vi "CSP_updateCSP_Parameters.vi"(8 "error in (no error)":errorcluster, 10 "Indicators Ref":T1, 11 "CSP.lvclass":refnum<class "CSP.lvclass">) -> (0 "error out":errorcluster, 3 "output cluster":refnum<class "CSP.lvclass">)   [LabVIEW 2016, in "Spatial Pattern Filter.lvlib" / "CSP.lvclass"]
uses:
  CSP.lvclass
  CSP.lvclass/CSP.ctl
  Spatial Pattern Filter.lvlib
panel:
  # "This VI is a part of BCI Design library, http://www.ru-bci.org \nCopyright © 2020, Sotnikov Peter, All rights reserved. License: GNU GPLv3"
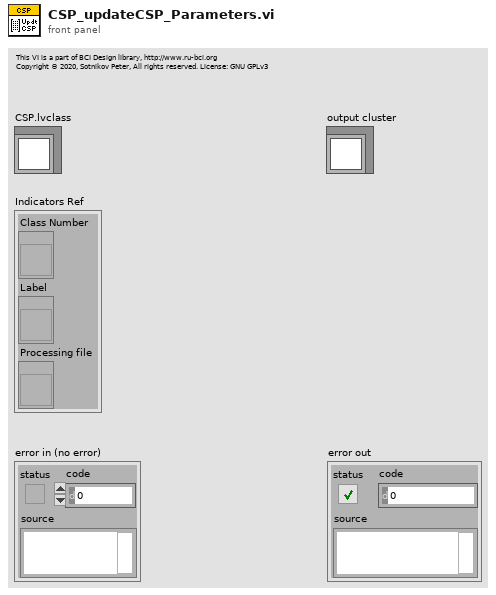
[diagram p1: front panel]
types:
  T1 = cluster{"Class Number":refnum<vi>, "Label":refnum<vi>, "Processing file":refnum<vi>}
  T2 = typedef "NI_Matrix.lvlib/RealMatrix.ctl" = dbl[][]
  T3 = cluster{"CSPMatrix":T2, "CovarianceMatrix1":T2, "CovarianceMatrix2":T2}[]
  T4 = cluster{"CSPMatrix":T2, "CovarianceMatrix1":T2, "CovarianceMatrix2":T2}
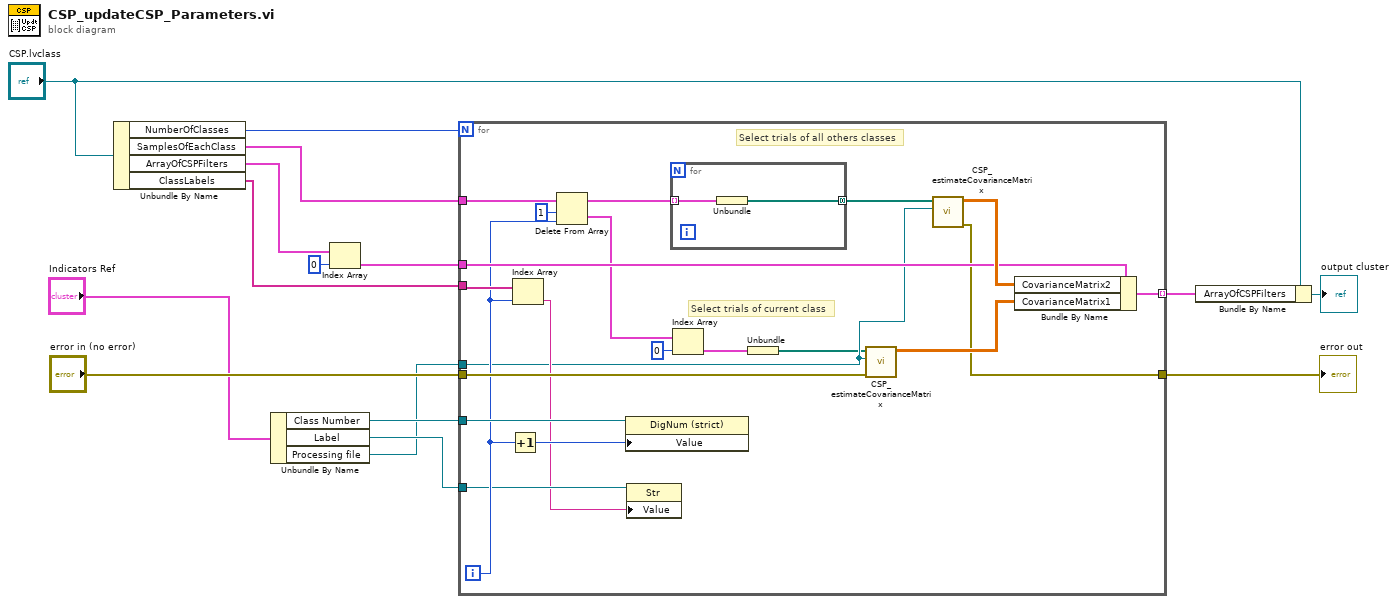
[diagram p0: block diagram]
diagram:
  n1 = Unbundle By Name("CSP.lvclass") -> ("NumberOfClasses"=w14:i32, "SamplesOfEachClass"=w15:cluster{"ArrayOfFiles":path[]}[], "ArrayOfCSPFilters"=w9:T3, "ClassLabels"=w3:string[])
  n2 = Unbundle By Name("Indicators Ref") -> ("Class Number"=w4:refnum<vi>, "Label"=w2:refnum<vi>, "Processing file"=w1:refnum<vi>)
  n3 = Index Array(array=w9, index=0) -> (element=w7:T4)
  n4 = for {
    N: w14 -> [_]
    tunnel: w15 -> [w32]
    tunnel: [w36] -> w6 mode=indexing
    tunnel: "error in (no error)" -> [w31]
    tunnel: [w27] -> w10
    tunnel: w7 -> [w30]
    tunnel: w4 -> [w26]
    tunnel: w3 -> [w24]
    tunnel: w2 -> [w22]
    tunnel: w1 -> [w20]
    i -> [w23]
    # "Select trials of current class"
    # "Select trials of all others classes"
    n5 = Increment(x=w23) -> (x+1=w25:i32)
    n6 = Index Array(array=w24, index=w23) -> (element=w21:string)
    n7 = Delete From Array(array=w32, length=1, index=w23) -> (deleted portion=w29:cluster{"ArrayOfFiles":path[]}[], array with subset deleted=w19:cluster{"ArrayOfFiles":path[]}[])
    n8 = property class="DigNum (strict)"(reference=w26, "Value"=w25) -> ()  [unwired: 1 in, 2 out]
    n9 = property class="Str"(reference=w22, "Value"=w21) -> ()  [unwired: 1 in, 2 out]
    n10 = for {
      tunnel: w19 -> [w38] mode=indexing
      tunnel: [w37] -> w18 mode=concatenating
      n11 = Unbundle(w38) -> ("ArrayOfFiles"=w37:path[])
    }
    n12 = Index Array(array=w29, index=0 ("index (row)")) -> (element=w17:cluster{"ArrayOfFiles":path[]})
    n13 = Unbundle(w17) -> ("ArrayOfFiles"=w16:path[])
    n14 = call "CSP_estimateCovarianceMatrix.vi"("error in (no error)"=w31, "Processing file"=w20, "FilePaths"=w16) -> ("Covariance Matrix"=w33:T2)  [unwired: 6 in, 2 out]
    n15 = call "CSP_estimateCovarianceMatrix.vi"("Processing file"=w20, "FilePaths"=w18) -> ("error out"=w27:errorcluster, "Covariance Matrix"=w34:T2)  [unwired: 7 in, 1 out]
    n16 = Bundle By Name(cluster=w30, "CovarianceMatrix2"=w34, "CovarianceMatrix1"=w33) -> (w36:T4)
  }
  "error out" <- w10
  n17 = Bundle By Name(cluster="CSP.lvclass", "ArrayOfCSPFilters"=w6) -> (→"output cluster":refnum<class "CSP.lvclass">)
